vi "Send SMS.vi"(5 "return address":string="hybridcryo@magnet.fsu.edu", 7 "smtp server":string="mail.magnet.fsu.edu", 9 "message":string="This is a test ", 10 "subject":string="Test SMS", 11 "Phone #":string="(asdf850)55asdf5-5555dsf") -> (0 "error out":errorcluster)   [LabVIEW 2025]
doc: "Author: Scott Hannahs <sth@magnet.fsu.edu>\n\nThis software is licensed for use under the “MIT License\"\nCopyright (c) 2025 Scott Hannahs, sth@sth@magnet.sthnet.net\n\nPermission is hereby granted, free of charge, to any person obtaining a copy of this software and associated documentation files (the \"Software\"), to deal in the Software without restriction, including without limitation the rights to use, copy, modify, merge, publish, distribute, sublicense, and/or sell copies of the Software, and to permit persons to whom the Software is furnished to do so, subject to the following conditions: The above copyright notice and this permission notice shall be included in all copies or substantial portions of the Software.\n\nTHE SOFTWARE IS PROVIDED \"AS IS\", WITHOUT WARRANTY OF ANY KIND, EXPRESS OR IMPLIED, INCLUDING BUT NOT LIMITED TO THE WARRANTIES OF MERCHANTABILITY, FITNESS FOR A PARTICULAR PURPOSE AND NONINFRINGEMENT. IN NO EVENT SHALL THE AUTHORS OR COPYRIGHT HOLDERS BE LIABLE FOR ANY CLAIM, DAMAGES OR OTHER LIABILITY, WHETHER IN AN ACTION OF CONTRACT, TORT OR OTHERWISE, ARISING FROM, OUT OF OR IN CONNECTION WITH THE SOFTWARE OR THE USE OR OTHER DEALINGS IN THE SOFTWARE."
uses:
  <vilib>/regexp/Match Regular Expression.xnode
  <vilib>/smtpClient/LabVIEWSMTPClient.lvlib
panel:
  # "Sends text message through 7 different providers.  Phone number must have 10 digits but can be any format."
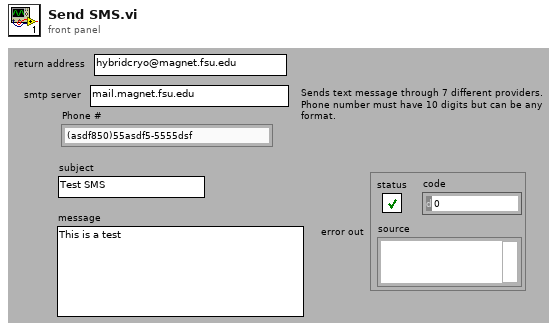
[diagram p1: front panel]
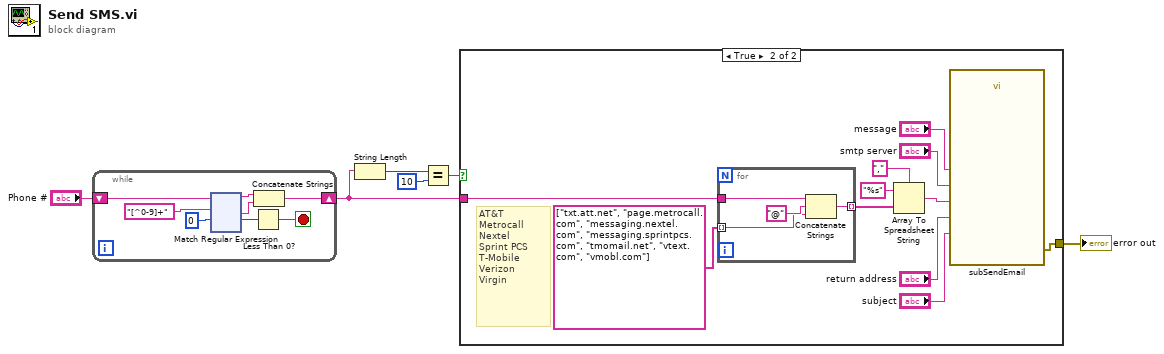
[diagram p0: block diagram]
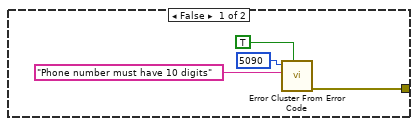
[diagram p2: hidden frame]
diagram:
  n1 = while {
    shift-right: [w12] -> w2
    shift-left: "Phone #" -> [w8]
    stop <- w13 stop-if-true
    n2 = xnode "Match Regular Expression"("input string"=w8, "regular expression"="[^0-9]+", "offset (0)"=0 ("offset past match")) -> ("before match"=w10:string, "after match"=w11:string, "offset past match"=w7:i32)  [unwired: 3 in, 2 out]
    n3 = Less Than 0?(x=w7) -> (x < 0?=w13:bool)
    n4 = Concatenate Strings(w10, w11) -> (w12:string)
  }
  n5 = String Length(string=w2) -> (length=w5:i32)
  n6 = Equal?(x=w5, y=10) -> (x = y?=w3:bool)
  n7 = case shown="True" w3 {
    tunnel: w2 -> [_ w145]
    tunnel: [w132 w143] -> w1
    frame False {
      n8 = call <vilib>:"Error Cluster From Error Code.vi"("show call chain? (False)"=TRUE, "error message (\"\")"="Phone number must have 10 digits" ("error message (\"\")"), "error code (0)"=5090) -> ("error out"=w132:errorcluster)  [unwired: 6 in]
    }
    frame True {
      # "AT&T\nMetrocall\nNextel\nSprint PCS\nT-Mobile\nVerizon\nVirgin"
      n9 = for {
        tunnel: string[] ["txt.att.net", "page.metrocall.com", "messaging.nextel.com", "messaging.sprintpcs.com", "tmomail.net", "vtext.com", "vmobl.com"] -> [w147] mode=indexing
        tunnel: w145 -> [w149]
        tunnel: [w148] -> w141 mode=indexing
        n10 = Concatenate Strings(w149, "@" ("string"), w147) -> (w148:string)
      }
      n11 = Array To Spreadsheet String(delimiter (Tab)=",", array=w141, 3:"%s" ("format string")) -> (spreadsheet string=w142:string)
      n12 = call <vilib>:"subSendEmail.vi"("Sender's Email Address"="return address", "Recipients"=w142, "Subject"="subject", "Message"="message", "Outgoing Mail Server (SMTP)"="smtp server") -> ("error out"=w143:errorcluster)  [unwired: 14 in]
    }
  }
  "error out" <- w1
